vi "Canwrite_jetson_L.vi"(10 "Param IN":T1) -> (2 "배열":T2(array[cluster]))   [LabVIEW 2019]
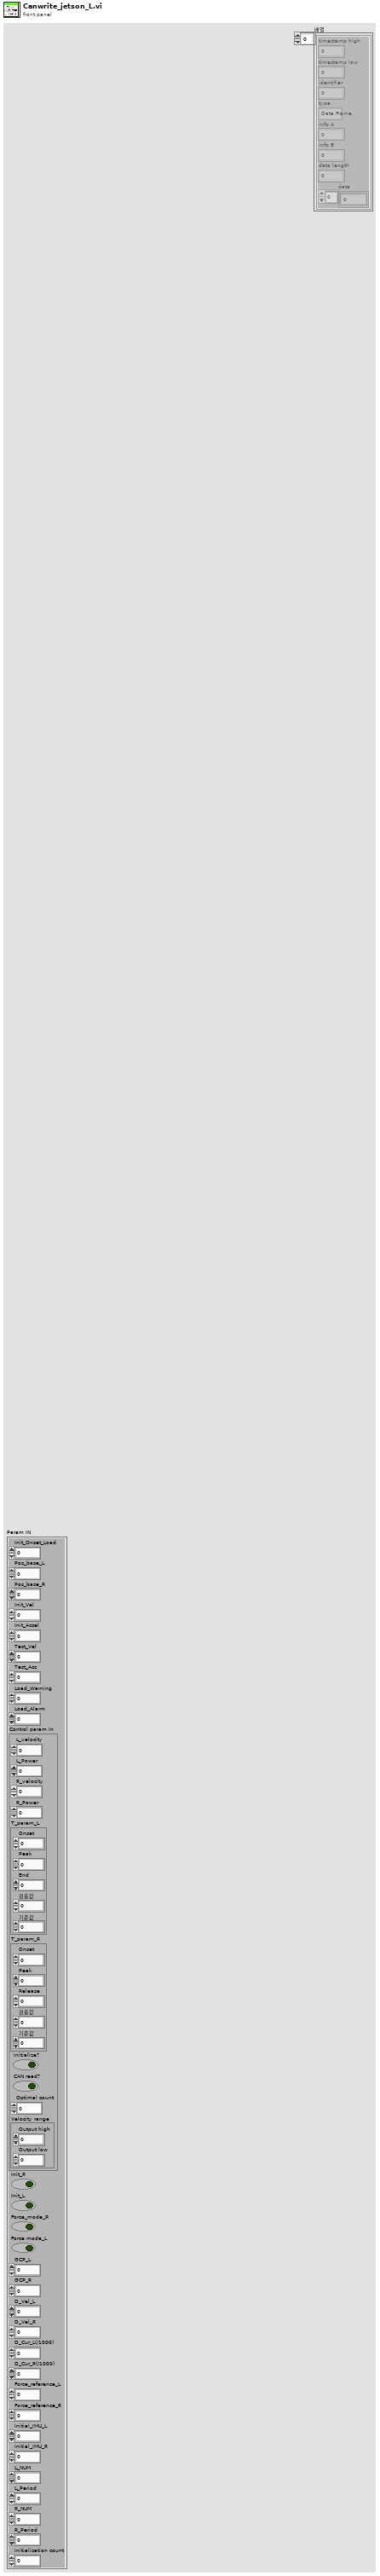
[diagram p1: front panel]
types:
  T1 = cluster{"Init_Onset_Load":sgl, "Pos_base_L":sgl, "Pos_base_R":sgl, "Init_Vel":i32, "Init_Accel":u32, "Test_Vel":i32, "Test_Acc":u32, "Load_Warning":sgl, "Load_Alarm":sgl, "Control param In":cluster{"L_velocity":u32, "L_Power":sgl, "R_velocity":u32, "R_Power":sgl, "T_param_L":cluster{"Onset":sgl, "Peak":sgl, "End":sgl, "검출값":sgl, "기준값":sgl}, "T_param_R":cluster{"Onset":sgl, "Peak":sgl, "Release":sgl, "검출값":sgl, "기준값":sgl}, "Initialize?":bool, "CAN read?":bool, "Optimal count":i32, "Velocity range":cluster{"Output high":dbl, "Output low":dbl}}, "Init_R":bool, "Init_L":bool, "Force_mode_R":bool, "Force mode_L":bool, "GCP_L":sgl, "GCP_R":sgl, "D_Vel_L":sgl, "D_Vel_R":sgl, "D_Cur_L(/1000)":sgl, "D_Cur_R(/1000)":sgl, "Force_reference_L":sgl, "Force_reference_R":sgl, "Initial_IMU_L":sgl, "Initial_IMU_R":sgl, "L_NUM":u32, "L_Period":i16, "R_NUM":u32, "R_Period":i16, "Initialization count":i32}
  T2 = cluster{"timestamp high":u32, "timestamp low":u32, "identifier":u32, "type":enum8{"Data Frame", "Remote Frame", "(reserved)", "(reserved) ", "(reserved)  ", "(reserved)   ", "Bus Error", "Transceiver Fault"}, "info A":u8, "info B":u8, "data length":u8, "data":u8[]}[]
  T3 = cluster{"timestamp high":u32, "timestamp low":u32, "identifier":u32, "type":enum8{"Data Frame", "Remote Frame", "(reserved)", "(reserved) ", "(reserved)  ", "(reserved)   ", "Bus Error", "Transceiver Fault"}, "info A":u8, "info B":u8, "data length":u8, "data":u8[]}
  T4 = enum8{"Data Frame", "Remote Frame", "(reserved)", "(reserved) ", "(reserved)  ", "(reserved)   ", "Bus Error", "Transceiver Fault"}
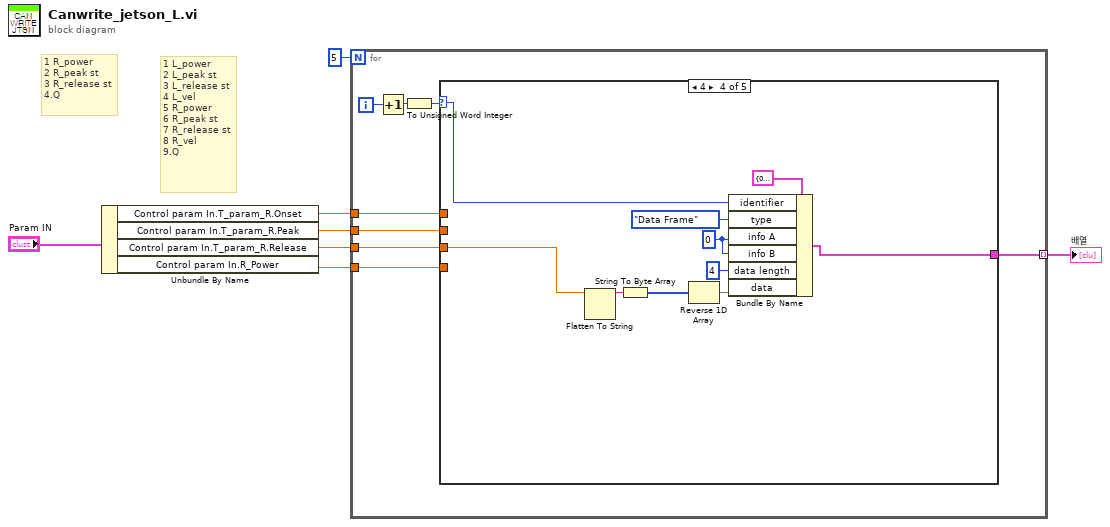
[diagram p0: block diagram]
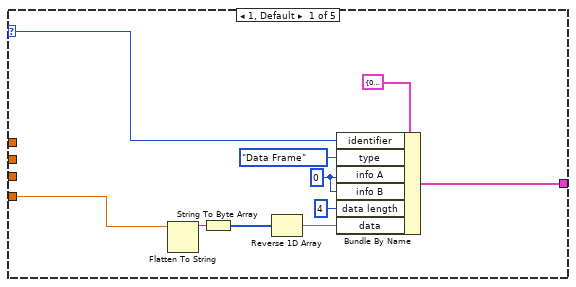
[diagram p2: hidden frame]
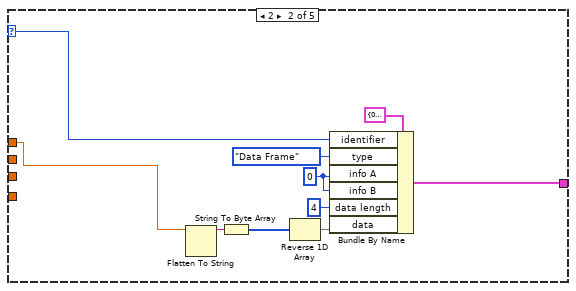
[diagram p3: hidden frame]
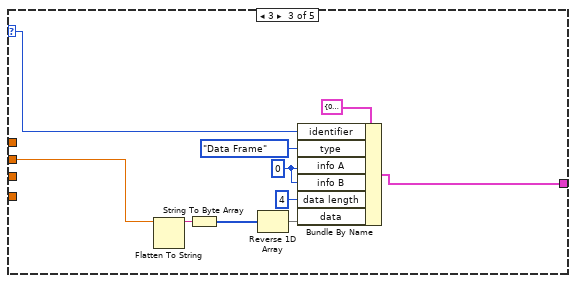
[diagram p4: hidden frame]
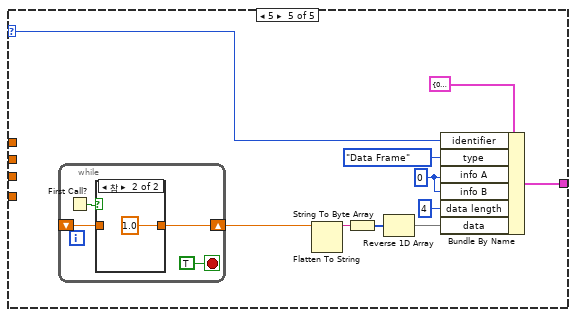
[diagram p5: hidden frame]
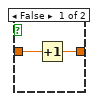
[diagram p6: hidden frame]
diagram:
  # "1 R_power\n2 R_peak st\n3 R_release st\n4.Q"
  # "1 L_power\n2 L_peak st\n3 L_release st\n4 L_vel\n5 R_power\n6 R_peak st\n7 R_release st\n8 R_vel\n9.Q"
  n1 = Unbundle By Name("Param IN") -> ("Control param In.T_param_R.Onset"=w2:sgl, "Control param In.T_param_R.Peak"=w6:sgl, "Control param In.T_param_R.Release"=w5:sgl, "Control param In.R_Power"=w4:sgl)
  n2 = for {
    N: 5 -> [_]
    tunnel: w6 -> [w15]
    tunnel: w5 -> [w14]
    tunnel: [w13] -> w3 mode=indexing
    tunnel: w4 -> [w9]
    tunnel: w2 -> [w8]
    i -> [w12]
    n3 = Increment(x=w12) -> (x+1=w11:i32)
    n4 = To Unsigned Word Integer(number=w11) -> (unsigned 16bit integer=w10:u16)
    n5 = case shown="4" w10 {
      selector: w10 -> [w18 w32 w38 w48 w58]
      tunnel: w15 -> [_ _ w36 _ _]
      tunnel: w14 -> [_ _ _ w46 _]
      tunnel: [w22 w31 w39 w49 w62] -> w13
      tunnel: w9 -> [w17 _ _ _ _]
      tunnel: w8 -> [_ w26 _ _ _]
      frame 1, Default {
        w24 = u8 0 ("info A")
        n6 = Flatten To String(anything=w17) -> (data string=w21:string)  [unwired: 3 in, 2 out]
        n7 = String To Byte Array(string=w21) -> (unsigned byte array=w20:u8[])
        n8 = Reverse 1D Array(array=w20) -> (reversed array=w19:u8[])
        n9 = Bundle By Name(cluster=T3 {"timestamp high"=0, "timestamp low"=0, "identifier"=0, "type"=enum."Data Frame", "info A"=0, "info B"=0, "data length"=0, "data"=[0, 0, 0, 0, 0, 0, 0, 0]} ("배열[0]"), "identifier"=w18, "type"=T4."Data Frame", "info A"=w24, "info B"=w24, "data length"=u8 4, "data"=w19) -> (w22:T3)
      }
      frame 2 {
        w34 = u8 0 ("info A")
        n10 = Flatten To String(anything=w26) -> (data string=w30:string)  [unwired: 3 in, 2 out]
        n11 = String To Byte Array(string=w30) -> (unsigned byte array=w29:u8[])
        n12 = Reverse 1D Array(array=w29) -> (reversed array=w28:u8[])
        n13 = Bundle By Name(cluster=T3 {"timestamp high"=0, "timestamp low"=0, "identifier"=0, "type"=enum."Data Frame", "info A"=0, "info B"=0, "data length"=0, "data"=[0, 0, 0, 0, 0, 0, 0, 0]} ("배열[0]"), "identifier"=w32, "type"=T4."Data Frame", "info A"=w34, "info B"=w34, "data length"=u8 4, "data"=w28) -> (w31:T3)
      }
      frame 3 {
        w44 = u8 0 ("info A")
        n14 = Flatten To String(anything=w36) -> (data string=w42:string)  [unwired: 3 in, 2 out]
        n15 = String To Byte Array(string=w42) -> (unsigned byte array=w41:u8[])
        n16 = Reverse 1D Array(array=w41) -> (reversed array=w40:u8[])
        n17 = Bundle By Name(cluster=T3 {"timestamp high"=0, "timestamp low"=0, "identifier"=0, "type"=enum."Data Frame", "info A"=0, "info B"=0, "data length"=0, "data"=[0, 0, 0, 0, 0, 0, 0, 0]} ("배열[0]"), "identifier"=w38, "type"=T4."Data Frame", "info A"=w44, "info B"=w44, "data length"=u8 4, "data"=w40) -> (w39:T3)
      }
      frame 4 {
        w54 = u8 0 ("info A")
        n18 = Flatten To String(anything=w46) -> (data string=w52:string)  [unwired: 3 in, 2 out]
        n19 = String To Byte Array(string=w52) -> (unsigned byte array=w51:u8[])
        n20 = Reverse 1D Array(array=w51) -> (reversed array=w50:u8[])
        n21 = Bundle By Name(cluster=T3 {"timestamp high"=0, "timestamp low"=0, "identifier"=0, "type"=enum."Data Frame", "info A"=0, "info B"=0, "data length"=0, "data"=[0, 0, 0, 0, 0, 0, 0, 0]} ("배열[0]"), "identifier"=w48, "type"=T4."Data Frame", "info A"=w54, "info B"=w54, "data length"=u8 4, "data"=w50) -> (w49:T3)
      }
      frame 5 {
        w64 = u8 0 ("info A")
        n22 = while {
          shift-right: [w67] -> w57
          shift-left: _ -> [w66]
          stop <- TRUE stop-if-true
          n23 = First Call?() -> (First Call?: T/F=w68:bool)
          n24 = case shown="참" w68 {
            tunnel: [w70 sgl 1.0] -> w67
            tunnel: w66 -> [w71 _]
            frame False {
              n25 = Increment(x=w71) -> (x+1=w70:sgl)
            }
            frame True {
            }
          }
        }
        n26 = Flatten To String(anything=w57) -> (data string=w61:string)  [unwired: 3 in, 2 out]
        n27 = String To Byte Array(string=w61) -> (unsigned byte array=w60:u8[])
        n28 = Reverse 1D Array(array=w60) -> (reversed array=w59:u8[])
        n29 = Bundle By Name(cluster=T3 {"timestamp high"=0, "timestamp low"=0, "identifier"=0, "type"=enum."Data Frame", "info A"=0, "info B"=0, "data length"=0, "data"=[0, 0, 0, 0, 0, 0, 0, 0]} ("배열[0]"), "identifier"=w58, "type"=T4."Data Frame", "info A"=w64, "info B"=w64, "data length"=u8 4, "data"=w59) -> (w62:T3)
      }
    }
  }
  "배열" <- w3
